vi "190625_Simulation_FreCTO_PC.vi"() -> ()   [LabVIEW 2019]
uses:
  <vilib>/Utility/file.llb/Read Delimited Spreadsheet (DBL).vi
panel:
  in  "X_Type":string(combo)="Notch15"
  in  "X_pole":string(combo)="4352"
  in  "Z_Type":string(combo)="Notch15"
  in  "Z_pole":string(combo)="4952"
  out "all time(s)":dbl
  out "Time slots (sec)":dbl[](array[numeric]) format="%#.10f"
  in  "Sample Rate (Hz)":dbl=1000.0 format="%#_13g"
  in  "STOP":bool
  in  "Load":bool
  in  "CLEAR":bool
  in  "RUN":bool
  out "RMS  X (um)":dbl format="%0.2f"
  out "MAX  X (um)":dbl format="%0.2f"
  out "RMS (one) X (um)":dbl format="%0.2f"
  out "Output X (mm)":dbl[](graph)
  out "CMD X (mm)":dbl[](graph)
  out "Position Error X (um)":dbl[](graph)
  out "Position Command X (mm)":dbl[](graph)
  out "time length":i32=15000
  out "start time":i32=7500
  out "RMS (one) Z (um)":dbl format="%0.2f"
  out "MAX  Z (um)":dbl format="%0.2f"
  out "RMS  Z (um)":dbl format="%0.2f"
  out "Position Error Z (um)":dbl[](graph)
  out "CMD Z (mm)":dbl[](graph)
  out "Output Z (mm)":dbl[](graph)
  out "Position Command Z (mm)":dbl[](graph)
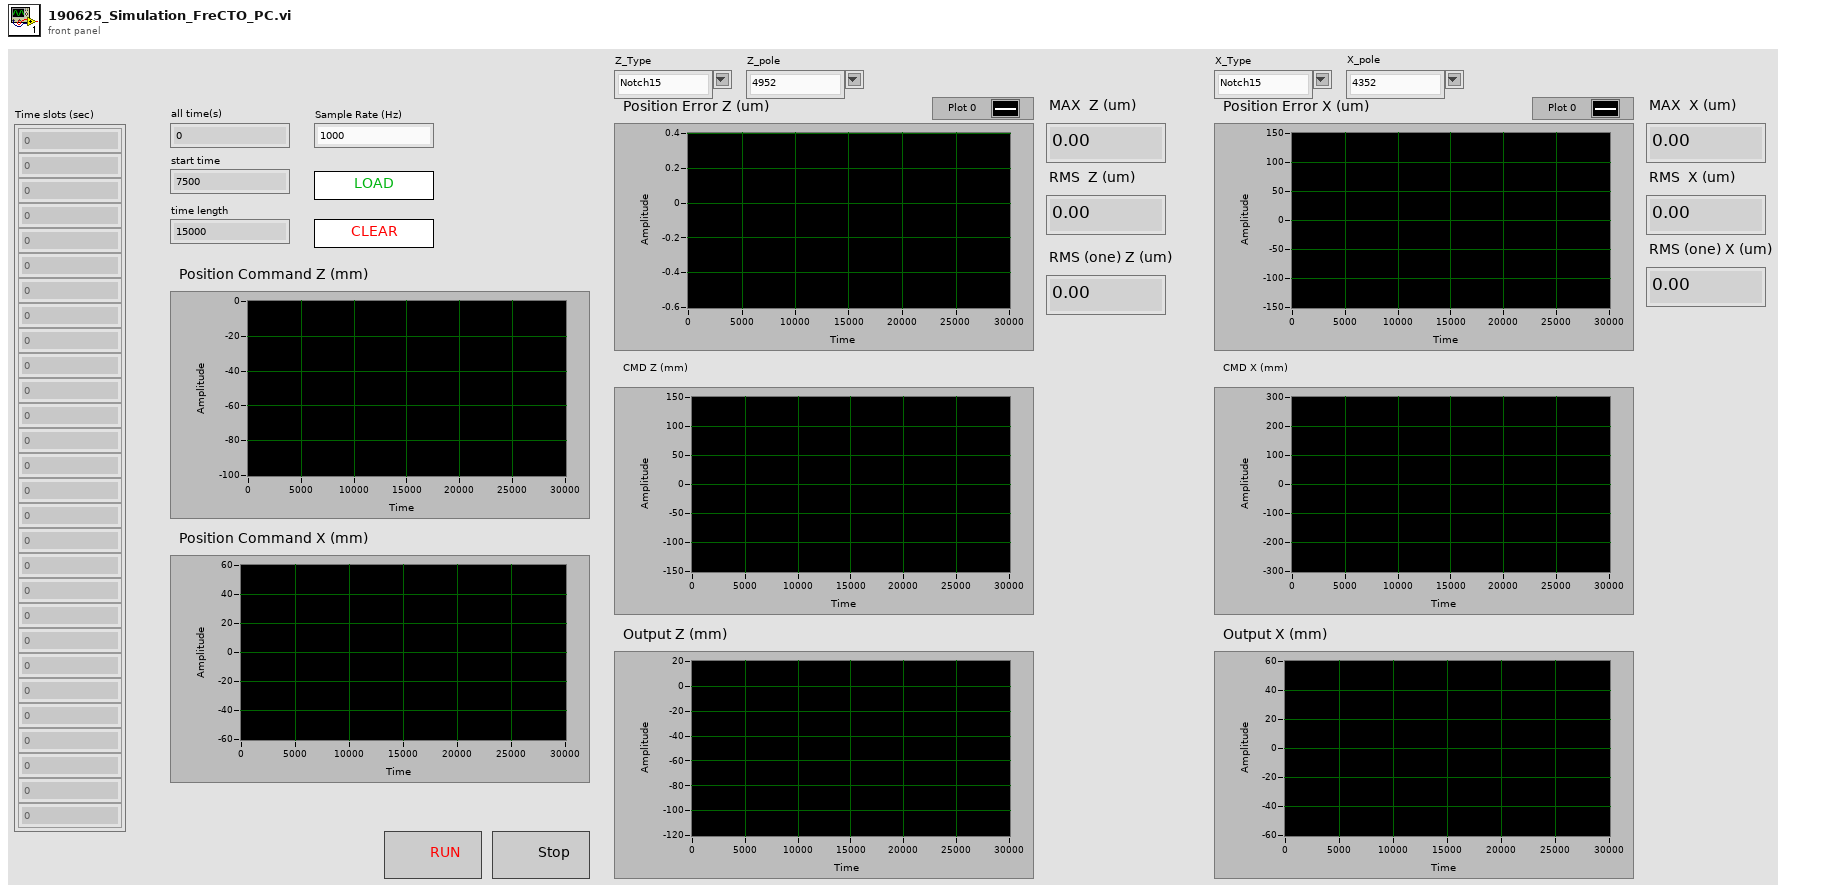
[diagram p1: front panel]
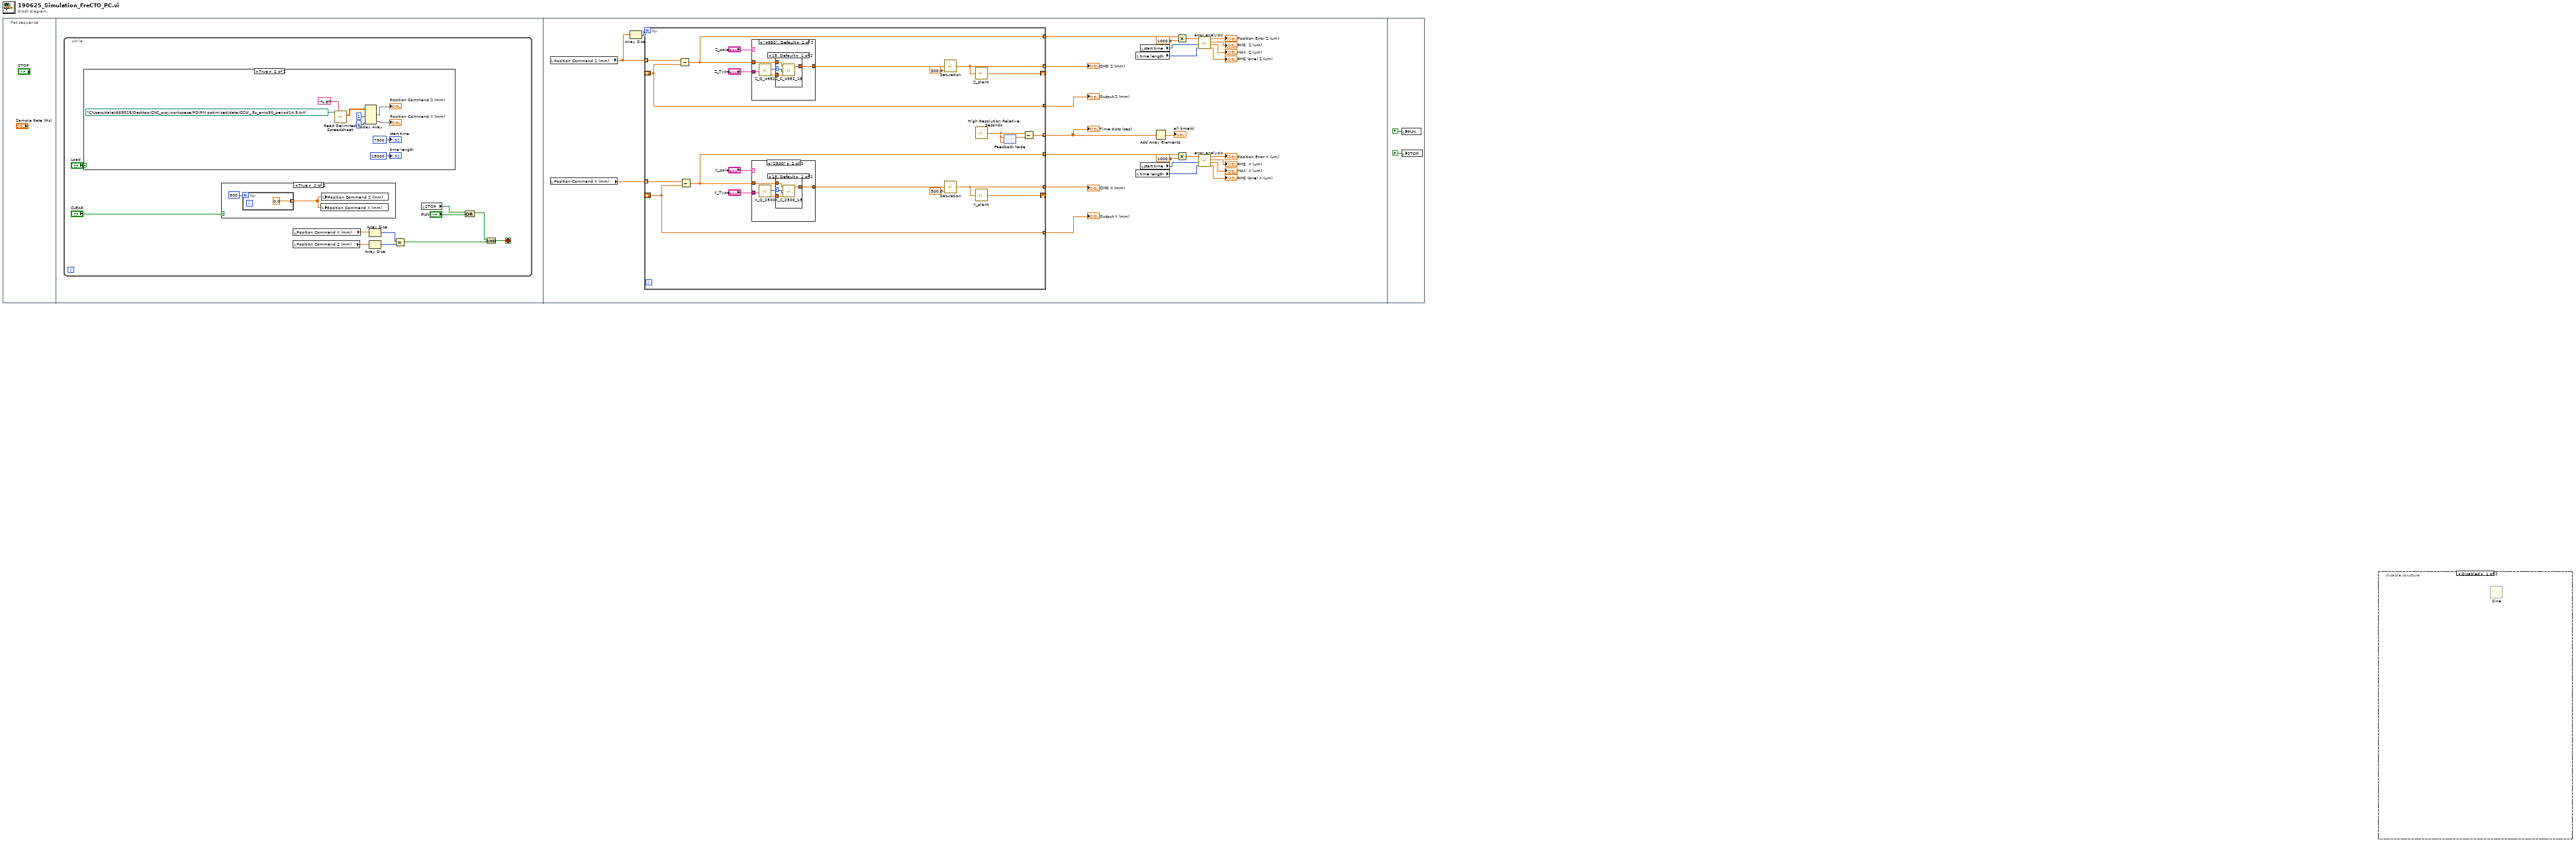
[diagram p0: block diagram]
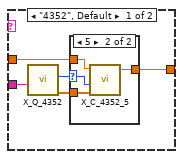
[diagram p4: hidden frame]
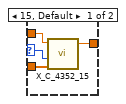
[diagram p5: hidden frame]
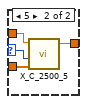
[diagram p6: hidden frame]
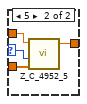
[diagram p7: hidden frame]
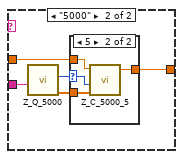
[diagram p8: hidden frame]
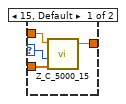
[diagram p9: hidden frame]
diagram:
  n1 = flat-sequence {
    frame #0 {
    }
    frame #1 {
      n2 = while {
        stop <- w8 stop-if-true
        n3 = case shown="True" "Load" {
          frame False {
          }
          frame True {
            n4 = call-poly <vilib>:"Read Delimited Spreadsheet.vi"("file path (dialog if empty)"=path "C:/Users/dalek669528/Desktop/CNC_proj/workspace/PDIPM optimized/data/CCW_.5s_amp50_period14.5.txt", "format (%.3f)"="%.8f") -> ("all rows"=w19:dbl[][])  [unwired: 8 in, 5 out]
            n5 = Index Array(array=w19, index (col) #1=1 ("disabled index (col)"), index (col) #2=0 ("index (col)")) -> (element #1=→"Position Command Z (mm)":dbl[], element #2=→"Position Command X (mm)":dbl[])  [unwired: 2 in]
            "start time" <- 7500 ("start time")
            "time length" <- 15000 ("time length")
          }
        }
        n6 = case shown="True" "CLEAR" {
          frame False {
          }
          frame True {
            n7 = for {
              N: 500 -> [_]
              tunnel: [0.0 ("element")] -> w13 mode=indexing
            }
            n8 = local write "Position Command X (mm)"(w13) -> ()
            n9 = local write "Position Command Z (mm)"(w13) -> ()
          }
        }
        n10 = local read "Position Command X (mm)"() -> (w9:dbl[])
        n11 = local read "Position Command Z (mm)"() -> (w10:dbl[])
        n12 = Array Size(array=w10) -> (size(s)=w6:i32)
        n13 = Array Size(array=w9) -> (size(s)=w7:i32)
        n14 = Equal?(x=w7, y=w6) -> (x = y?=w5:bool)
        n15 = local read "STOP"() -> (w1:bool)
        n16 = Compound Arithmetic op=OR(w1, "RUN") -> (w3:bool)
        n17 = And(x=w3, y=w5) -> (x .and. y?=w8:bool)
      }
    }
    frame #2 {
      n18 = local read "Position Command Z (mm)"() -> (w49:dbl[])
      n19 = local read "Position Command X (mm)"() -> (w33:dbl[])
      n20 = Array Size(array=w49) -> (size(s)=w48:i32)
      n21 = for {
        N: w48 -> [_]
        shift-right: [w65] -> _
        shift-left: _ -> [w60]
        tunnel: [w60] -> w24 mode=indexing
        tunnel: [w57] -> w29 mode=indexing
        tunnel: [w64] -> w50 mode=indexing
        tunnel: w49 -> [w62] mode=indexing
        tunnel: w33 -> [w61] mode=indexing
        shift-right: [w66] -> _
        shift-left: _ -> [w52]
        tunnel: [w67] -> w32 mode=indexing
        tunnel: [w54] -> w27 mode=indexing
        tunnel: [w52] -> w25 mode=indexing
        tunnel: [w68] -> w31 mode=indexing
        n22 = Subtract(x=w62, y=w60) -> (x-y=w57:dbl)
        n23 = Subtract(x=w61, y=w52) -> (x-y=w54:dbl)
        n24 = case shown="\"4952\", Default" "Z_pole" {
          tunnel: "Z_Type" -> [w102 w115]
          tunnel: w57 -> [w99 w112]
          tunnel: [w98 w111] -> w56
          frame "4952", Default {
            n25 = call "Z_Q_4952.vi"("Type"=w102) -> ("Qn"=w100:dbl[], "L"=w101:i32)  [unwired: 9 in]
            n26 = case shown="15, Default" w101 {
              selector: w101 -> [w104 w108]
              tunnel: w100 -> [w103 w107]
              tunnel: w99 -> [w106 w110]
              tunnel: [w105 w109] -> w98
              frame 15, Default {
                n27 = call "Z_C_4952_15.vi"("ek"=w106, "length"=w104, "q"=w103) -> ("uk"=w105:dbl)  [unwired: 4 in]
              }
              frame 5 {
                n28 = call "Z_C_4952_5.vi"("ek"=w110, "length"=w108, "q"=w107) -> ("uk"=w109:dbl)  [unwired: 4 in]
              }
            }
          }
          frame "5000" {
            n29 = call "Z_Q_5000.vi"("Type"=w115) -> ("Qn"=w113:dbl[], "L"=w114:i32)  [unwired: 9 in]
            n30 = case shown="5" w114 {
              selector: w114 -> [w117 w121]
              tunnel: w113 -> [w116 w120]
              tunnel: w112 -> [w119 w123]
              tunnel: [w118 w122] -> w111
              frame 15, Default {
                n31 = call "Z_C_5000_15.vi"("ek"=w119, "length"=w117, "q"=w116) -> ("uk"=w118:dbl)  [unwired: 4 in]
              }
              frame 5 {
                n32 = call "Z_C_5000_5.vi"("ek"=w123, "length"=w121, "q"=w120) -> ("uk"=w122:dbl)  [unwired: 4 in]
              }
            }
          }
        }
        n33 = case shown="\"2500\"" "X_pole" {
          tunnel: "X_Type" -> [w76 w89]
          tunnel: w54 -> [w73 w86]
          tunnel: [w72 w85] -> w53
          frame "4352", Default {
            n34 = call "X_Q_4352.vi"("Type"=w76) -> ("Qn"=w74:dbl[], "L"=w75:i32)  [unwired: 9 in]
            n35 = case shown="5" w75 {
              selector: w75 -> [w78 w82]
              tunnel: w74 -> [w77 w81]
              tunnel: w73 -> [w80 w84]
              tunnel: [w79 w83] -> w72
              frame 15, Default {
                n36 = call "X_C_4352_15.vi"("ek"=w80, "length"=w78, "q"=w77) -> ("uk"=w79:dbl)  [unwired: 4 in]
              }
              frame 5 {
                n37 = call "X_C_4352_5.vi"("ek"=w84, "length"=w82, "q"=w81) -> ("uk"=w83:dbl)  [unwired: 4 in]
              }
            }
          }
          frame "2500" {
            n38 = call "X_Q_2500.vi"("Type"=w89) -> ("Qn"=w87:dbl[], "L"=w88:i32)  [unwired: 9 in]
            n39 = case shown="15, Default" w88 {
              selector: w88 -> [w91 w95]
              tunnel: w87 -> [w90 w94]
              tunnel: w86 -> [w93 w97]
              tunnel: [w92 w96] -> w85
              frame 15, Default {
                n40 = call "X_C_2500_15.vi"("ek"=w93, "length"=w91, "q"=w90) -> ("uk"=w92:dbl)  [unwired: 4 in]
              }
              frame 5 {
                n41 = call "X_C_2500_5.vi"("ek"=w97, "length"=w95, "q"=w94) -> ("uk"=w96:dbl)  [unwired: 4 in]
              }
            }
          }
        }
        n42 = call "Saturation.vi"("Vmax"=300.0, "uk"=w56) -> ("real uk"=w64:dbl)  [unwired: 3 in]
        n43 = call "Saturation.vi"("Vmax"=300.0, "uk"=w53) -> ("real uk"=w67:dbl)  [unwired: 3 in]
        n44 = call "Z_plant.vi"("u"=w64) -> ("y"=w65:dbl)  [unwired: 4 in]
        n45 = call <vilib>:"High Resolution Relative Seconds.vi"() -> ("relative seconds"=w63:dbl)
        n46 = call "X_plant.vi"("u"=w67) -> ("y"=w66:dbl)  [unwired: 4 in]
        n47 = feedback #1(w63) -> (w69:dbl)
        n48 = feedback-in #1(w63) -> ()
        n49 = Subtract(x=w63, y=w69) -> (x-y=w68:dbl)
      }
      "Output Z (mm)" <- w24
      "CMD Z (mm)" <- w50
      "Output X (mm)" <- w25
      "CMD X (mm)" <- w32
      "Time slots (sec)" <- w31
      n50 = local read "time length"() -> (w43:i32)
      n51 = local read "time length"() -> (w37:i32)
      n52 = local read "start time"() -> (w42:i32)
      n53 = local read "start time"() -> (w36:i32)
      n54 = Add Array Elements(numeric array=w31) -> (sum=→"all time(s)":dbl)
      n55 = Multiply(x=w29, y=1000.0) -> (x*y=w41:dbl[])
      n56 = Multiply(x=w27, y=1000.0) -> (x*y=w34:dbl[])
      n57 = call "error_analysis.vi"("tLength"=w43, "t0"=w42, "data in (um)"=w41) -> ("rms (one) (um)"=→"RMS (one) Z (um)":dbl, "max err (um)"=→"MAX  Z (um)":dbl, "rms (all) (um)"=→"RMS  Z (um)":dbl, "data out (um)"=→"Position Error Z (um)":dbl[])  [unwired: 5 in]
      n58 = call "error_analysis.vi"("tLength"=w37, "t0"=w36, "data in (um)"=w34) -> ("rms (one) (um)"=→"RMS (one) X (um)":dbl, "max err (um)"=→"MAX  X (um)":dbl, "rms (all) (um)"=→"RMS  X (um)":dbl, "data out (um)"=→"Position Error X (um)":dbl[])  [unwired: 5 in]
    }
    frame #3 {
      n59 = local write "RUN"(FALSE ("RUN")) -> ()
      n60 = local write "STOP"(FALSE ("STOP")) -> ()
    }
  }
  n61 = disable-structure shown="Disabled" {
    frame Disabled {
      n62 = Sine() -> ()  [unwired: 1 in, 1 out]
    }
    frame Enabled {
    }
  }
